vi "GraderMain.vi"   [LabVIEW 2015]
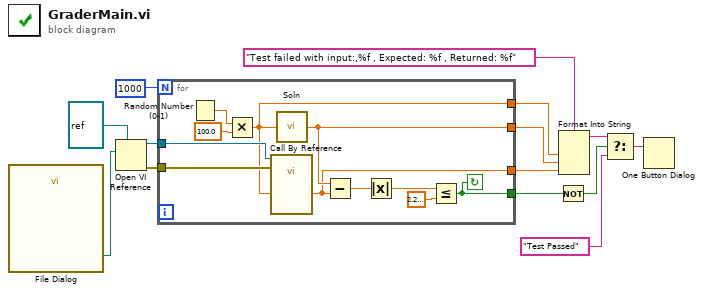
[diagram p0: block diagram]
diagram:
  n1 = call "File Dialog"() -> ("selected path"=w14:path)  [unwired: 12 in, 3 out]
  n2 = Open VI Reference(type specifier VI Refnum (for type only)=refnum<vi> refnum, vi path=w14) -> (vi reference=w11:refnum<vi>, error out=w10:errorcluster)  [unwired: 4 in]
  n3 = for {
    N: 1000 -> [_]
    tunnel: w11 -> [w25]
    tunnel: w10 -> [w24]
    tunnel: [w15] -> w6
    tunnel: [w21] -> w5
    tunnel: [w20] -> w4
    tunnel: [w16] -> w2
    stop <- w16 continue-if-true
    n4 = Random Number (0-1)() -> (number: 0 to 1=w23:dbl)
    n5 = Multiply(x=w23, y=100.0) -> (x*y=w15:dbl)
    n6 = call-by-ref "?"(reference=w25, error in=w24, "Celsius"=w15) -> ("Fahrenheit"=w20:dbl)  [unwired: 2 out]
    n7 = call "Soln.vi"("Celsius"=w15) -> ("Fahrenheit"=w21:dbl)
    n8 = Subtract(x=w21, y=w20) -> (x-y=w19:dbl)
    n9 = Absolute Value(x=w19) -> (abs(x)=w18:dbl)
    n10 = Less Or Equal?(x=w18, y=2.220446049250313e-16) -> (x <= y?=w16:bool)
  }
  n11 = Not(x=w2) -> (.not. x?=w1:bool)
  n12 = Format Into String(format string="Test failed with input:,%f , Expected: %f , Returned: %f", w6, w5, w4) -> (resulting string=w3:string)  [unwired: 2 in, 1 out]
  n13 = Select(t=w3, s=w1, f="Test Passed") -> (s? t:f=w8:string)
  n14 = One Button Dialog(message=w8) -> ()  [unwired: 1 in, 1 out]
